vi "Update GUI (SubVI).vi"(11 "Data out":T1={"VI References"=[], "Addresses"=[], "Pilot"=FALSE, "DO Data"=[], "Access Restricted?"=FALSE, "Pilot Control References"=[], "CoPilot Control References"=[], "cRIO Config"=[], "datalog Q"=refnum, "PS_P"={"AI"=[], "DI"=[], "DO"=[], "Serial"=[], "CPU"={"Total Load"=[], "Interrupt Load"=[], "Total Physical"=0.0, "Free Physical"=0.0, "Primary Disk Capacity"=0.0, "Primary Disk Free"=0.0}, "Stop"=FALSE, "DO Channel"=[]}, "PS_S"={"AI"=[], "DI"=[], "DO"=[], "Serial"=[], "CPU"={"Total Load"=[], "Interrupt Load"=[], "Total Physical"=0.0, "Free Physical"=0.0, "Primary Disk Capacity"=0.0, "Primary Disk Free"=0.0}, "Stop"=FALSE, "DO Channel"=[]}, "IDE_P"={"AI"=[], "DI"=[], "DO"=[], "Serial"=[], "CPU"={"Total Load"=[], "Interrupt Load"=[], "Total Physical"=0.0, "Free Physical"=0.0, "Primary Disk Capacity"=0.0, "Primary Disk Free"=0.0}, "Stop"=FALSE, "DO Channel"=[]}, "IDE_S"={"AI"=[], "DI"=[], "DO"=[], "Serial"=[], "CPU"={"Total Load"=[], "Interrupt Load"=[], "Total Physical"=0.0, "Free Physical"=0.0, "Primary Disk Capacity"=0.0, "Primary Disk Free"=0.0}, "Stop"=FALSE, "DO Channel"=[]}, "PDE_P"={"AI"=[], "DI"=[], "DO"=[], "Serial"=[], "CPU"={"Total Load"=[], "Interrupt Load"=[], "Total Physical"=0.0, "Free Physical"=0.0, "Primary Disk Capacity"=0.0, "Primary Disk Free"=0.0}, "Stop"=FALSE, "DO Channel"=[]}, "PDE_S"={"AI"=[], "DI"=[], "DO"=[], "Serial"=[], "CPU"={"Total Load"=[], "Interrupt Load"=[], "Total Physical"=0.0, "Free Physical"=0.0, "Primary Disk Capacity"=0.0, "Primary Disk Free"=0.0}, "Stop"=FALSE, "DO Channel"=[]}, "GUI References"={"Control Names"=[], "Control References"=[]}, "GUI Data"=[], "TCP - Serial"=[], "TCP-Serial Q"=refnum, "TCP Serial Ref"=[], "Data Sets"=[], "Last Data"=[], "Alarm Data"=[], "DI Data"=[], "Ack Data"=[], "Buzzer Data"=[], "Pilot DO"=[], "Co-Pilot DO"=[], "System Down?"=FALSE, "Log Data"=[], "Update Array"=[], "MCC Data Log"=[], "MCC Data Not"=refnum, "Thruster control"=[refnum, refnum, refnum, refnum, refnum, refnum, refnum, refnum, refnum], "waga notifier out"=refnum, "Wago  log"=[], "Thruster Cont"=[0.0, 0.0, 0.0, 0.0, 0.0, 0.0, 0.0, 0.0, 0.0], "Cam Cont"=[FALSE, FALSE, FALSE, FALSE, FALSE, TRUE], "PDE_P TH Cont"={"COM 10"=0.0, "COM 11"=0.0, "COM 12"=0.0, "COM 13"=0.0}, "PDE_S TH Cont"={"COM 10"=0.0, "COM 11"=0.0, "COM 12"=0.0, "COM 13"=0.0}} {"cRIO Config"."AI"."Interface Data"."Timing"."sample mode" items=["Finite Samples"=10178, "Continuous Samples"=10123, "Hardware Timed Single Point"=12522]; "cRIO Config"."Async"."Interface Data"."Data"."Minor Frame Count" min=5 max=8 step=1}) -> (3 "Data out":T1={"VI References"=[], "Addresses"=[], "Pilot"=FALSE, "DO Data"=[], "Access Restricted?"=FALSE, "Pilot Control References"=[], "CoPilot Control References"=[], "cRIO Config"=[], "datalog Q"=refnum, "PS_P"={"AI"=[], "DI"=[], "DO"=[], "Serial"=[], "CPU"={"Total Load"=[], "Interrupt Load"=[], "Total Physical"=0.0, "Free Physical"=0.0, "Primary Disk Capacity"=0.0, "Primary Disk Free"=0.0}, "Stop"=FALSE, "DO Channel"=[]}, "PS_S"={"AI"=[], "DI"=[], "DO"=[], "Serial"=[], "CPU"={"Total Load"=[], "Interrupt Load"=[], "Total Physical"=0.0, "Free Physical"=0.0, "Primary Disk Capacity"=0.0, "Primary Disk Free"=0.0}, "Stop"=FALSE, "DO Channel"=[]}, "IDE_P"={"AI"=[], "DI"=[], "DO"=[], "Serial"=[], "CPU"={"Total Load"=[], "Interrupt Load"=[], "Total Physical"=0.0, "Free Physical"=0.0, "Primary Disk Capacity"=0.0, "Primary Disk Free"=0.0}, "Stop"=FALSE, "DO Channel"=[]}, "IDE_S"={"AI"=[], "DI"=[], "DO"=[], "Serial"=[], "CPU"={"Total Load"=[], "Interrupt Load"=[], "Total Physical"=0.0, "Free Physical"=0.0, "Primary Disk Capacity"=0.0, "Primary Disk Free"=0.0}, "Stop"=FALSE, "DO Channel"=[]}, "PDE_P"={"AI"=[], "DI"=[], "DO"=[], "Serial"=[], "CPU"={"Total Load"=[], "Interrupt Load"=[], "Total Physical"=0.0, "Free Physical"=0.0, "Primary Disk Capacity"=0.0, "Primary Disk Free"=0.0}, "Stop"=FALSE, "DO Channel"=[]}, "PDE_S"={"AI"=[], "DI"=[], "DO"=[], "Serial"=[], "CPU"={"Total Load"=[], "Interrupt Load"=[], "Total Physical"=0.0, "Free Physical"=0.0, "Primary Disk Capacity"=0.0, "Primary Disk Free"=0.0}, "Stop"=FALSE, "DO Channel"=[]}, "GUI References"={"Control Names"=[], "Control References"=[]}, "GUI Data"=[], "TCP - Serial"=[], "TCP-Serial Q"=refnum, "TCP Serial Ref"=[], "Data Sets"=[], "Last Data"=[], "Alarm Data"=[], "DI Data"=[], "Ack Data"=[], "Buzzer Data"=[], "Pilot DO"=[], "Co-Pilot DO"=[], "System Down?"=FALSE, "Log Data"=[], "Update Array"=[], "MCC Data Log"=[], "MCC Data Not"=refnum, "Thruster control"=[refnum, refnum, refnum, refnum, refnum, refnum, refnum, refnum, refnum], "waga notifier out"=refnum, "Wago  log"=[], "Thruster Cont"=[0.0, 0.0, 0.0, 0.0, 0.0, 0.0, 0.0, 0.0, 0.0], "Cam Cont"=[FALSE, FALSE, FALSE, FALSE, FALSE, TRUE], "PDE_P TH Cont"={"COM 10"=0.0, "COM 11"=0.0, "COM 12"=0.0, "COM 13"=0.0}, "PDE_S TH Cont"={"COM 10"=0.0, "COM 11"=0.0, "COM 12"=0.0, "COM 13"=0.0}} {"cRIO Config"."AI"."Interface Data"."Timing"."sample mode" items=["Finite Samples"=10178, "Continuous Samples"=10123, "Hardware Timed Single Point"=12522]; "cRIO Config"."Async"."Interface Data"."Data"."Minor Frame Count" min=5 max=8 step=1})   [LabVIEW 2021]
doc: "output from the c-RIO will be updated here with the help of the 2D string array mapping from the intilizle array. based on the mapping teh index of the controls will be got and its match with the reference index and data will be updated"
uses:
  Controls/Host - GUI Data Cluster.ctl
  Analog Output/Controls/AO JSON Data Cluster.ctl
  Analog Output/Controls/AO Interface Data Cluster.ctl
  Analog Output/Controls/AO Channel Configuration Cluster.ctl
  Analog Output/Controls/AO Timing Cluster.ctl
  Digital Output/Controls/DIO Configuration cluster.ctl
  Digital Output/Controls/DIO Interface Data.ctl
  Digital Output/SubVIs/Digital Dynamic Cluster.ctl
  Async JSON Cluster.ctl
  Async Interface Data Cluster.ctl
  Async Serial/Controls/Async Serial Configuration Cluster.ctl
  Async Serial/Controls/Async Frame Info Cluster.ctl
  Async Serial/Controls/Async Message Info Cluster.ctl
  Controls/Host Data Cluster.ctl
  Main Engine/Controls/Main Engine CPU Info.ctl
panel:
  out "error out 2":errorcluster
  out "error out":errorcluster
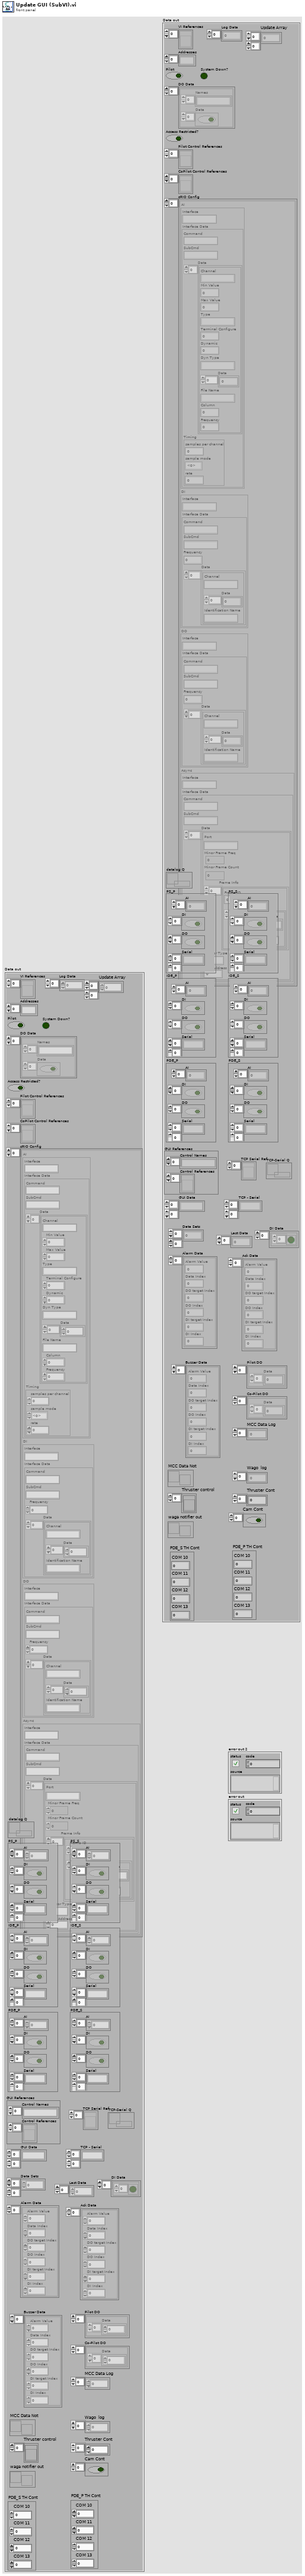
[diagram p1: front panel]
types:
  T1 = typedef "Host - GUI Data Cluster.ctl" = cluster{"VI References":refnum<vi>[], "Addresses":string[], "Pilot":bool, "DO Data":cluster{"Names":string[], "Data":bool[]}[], "Access Restricted?":bool, "Pilot Control References":refnum<vi>[], "CoPilot Control References":refnum<vi>[], "cRIO Config":cluster{"AI":T2, "DI":T6, "DO":T6, "Async":T9}[], "datalog Q":refnum<queue>, "PS_P":T14, "PS_S":T14, "IDE_P":T14, "IDE_S":T14, "PDE_P":T14, "PDE_S":T14, "GUI References":cluster{"Control Names":string[], "Control References":refnum<vi>[]}, "GUI Data":string[][], "TCP - Serial":string[][], "TCP-Serial Q":refnum<queue>, "TCP Serial Ref":refnum<vi>[], "Data Sets":dbl[][], "Last Data":dbl[], "Alarm Data":cluster{"Alarm Value":dbl, "Data Index":i32, "DO target Index":i32, "DO Index":i32, "DI target Index":i32, "DI Index":i32}[], "DI Data":cluster{bool[]}[], "Ack Data":cluster{"Alarm Value":dbl, "Data Index":i32, "DO target Index":i32, "DO Index":i32, "DI target Index":i32, "DI Index":i32}[], "Buzzer Data":cluster{"Alarm Value":dbl, "Data Index":i32, "DO target Index":i32, "DO Index":i32, "DI target Index":i32, "DI Index":i32}[], "Pilot DO":cluster{"Data":i32[]}[], "Co-Pilot DO":cluster{"Data":i32[]}[], "System Down?":bool, "Log Data":dbl[], "Update Array":i32[][], "MCC Data Log":dbl[], "MCC Data Not":refnum<notifier>, "Thruster control":refnum<vi>[], "waga notifier out":refnum<notifier>, "Wago  log":sgl[], "Thruster Cont":dbl[], "Cam Cont":bool[], "PDE_P TH Cont":cluster{"COM 10":dbl, "COM 11":dbl, "COM 12":dbl, "COM 13":dbl}, "PDE_S TH Cont":cluster{"COM 10":dbl, "COM 11":dbl, "COM 12":dbl, "COM 13":dbl}}
  T2 = typedef "AO JSON Data Cluster.ctl" = cluster{"Interface":string, "Interface Data":T3}
  T3 = typedef "AO Interface Data Cluster.ctl" = cluster{"Command":string, "SubCmd":string, "Data":T4[], "Timing":T5}
  T4 = typedef "AO Channel Configuration Cluster.ctl" = cluster{"Channel":string, "Min Value":dbl, "Max Value":dbl, "Type":string, "Terminal Configure":u16, "Dynamic":u8, "Dyn Type":string, "Data":dbl[], "File Name":string, "Column":i32, "Frequency":dbl}
  T5 = typedef "AO Timing Cluster.ctl" = cluster{"samples per channel":i32, "sample mode":i32, "rate":dbl}
  T6 = typedef "DIO Configuration cluster.ctl" = cluster{"Interface":string, "Interface Data":T7}
  T7 = typedef "DIO Interface Data.ctl" = cluster{"Command":string, "SubCmd":string, "Frequency":u16, "Data":T8[]}
  T8 = typedef "Digital Dynamic Cluster.ctl" = cluster{"Channel":string, "Data":u8[], "Identification Name":string}
  T9 = typedef "Async JSON Cluster.ctl" = cluster{"Interface":string, "Interface Data":T10}
  T10 = typedef "Async Interface Data Cluster.ctl" = cluster{"Command":string, "SubCmd":string, "Data":T11[]}
  T11 = typedef "Async Serial Configuration Cluster.ctl" = cluster{"Port":string, "Minor Frame Freq":u16, "Minor Frame Count":u16, "Frame Info":T12[], "Sensor Type":u16, "OIM Address":u16}
  T12 = typedef "Async Frame Info Cluster.ctl" = cluster{"Frame ID":u16, "Message Info":T13[]}
  T13 = typedef "Async Message Info Cluster.ctl" = cluster{"Message":u8[], "Message Name":string}
  T14 = typedef "Host Data Cluster.ctl" = cluster{"AI":dbl[], "DI":bool[], "DO":bool[], "Serial":string[][], "CPU":T15, "Stop":bool, "DO Channel":string[]}
  T15 = typedef "Main Engine CPU Info.ctl" = cluster{"Total Load":u32[], "Interrupt Load":u32[], "Total Physical":dbl, "Free Physical":dbl, "Primary Disk Capacity":dbl, "Primary Disk Free":dbl}
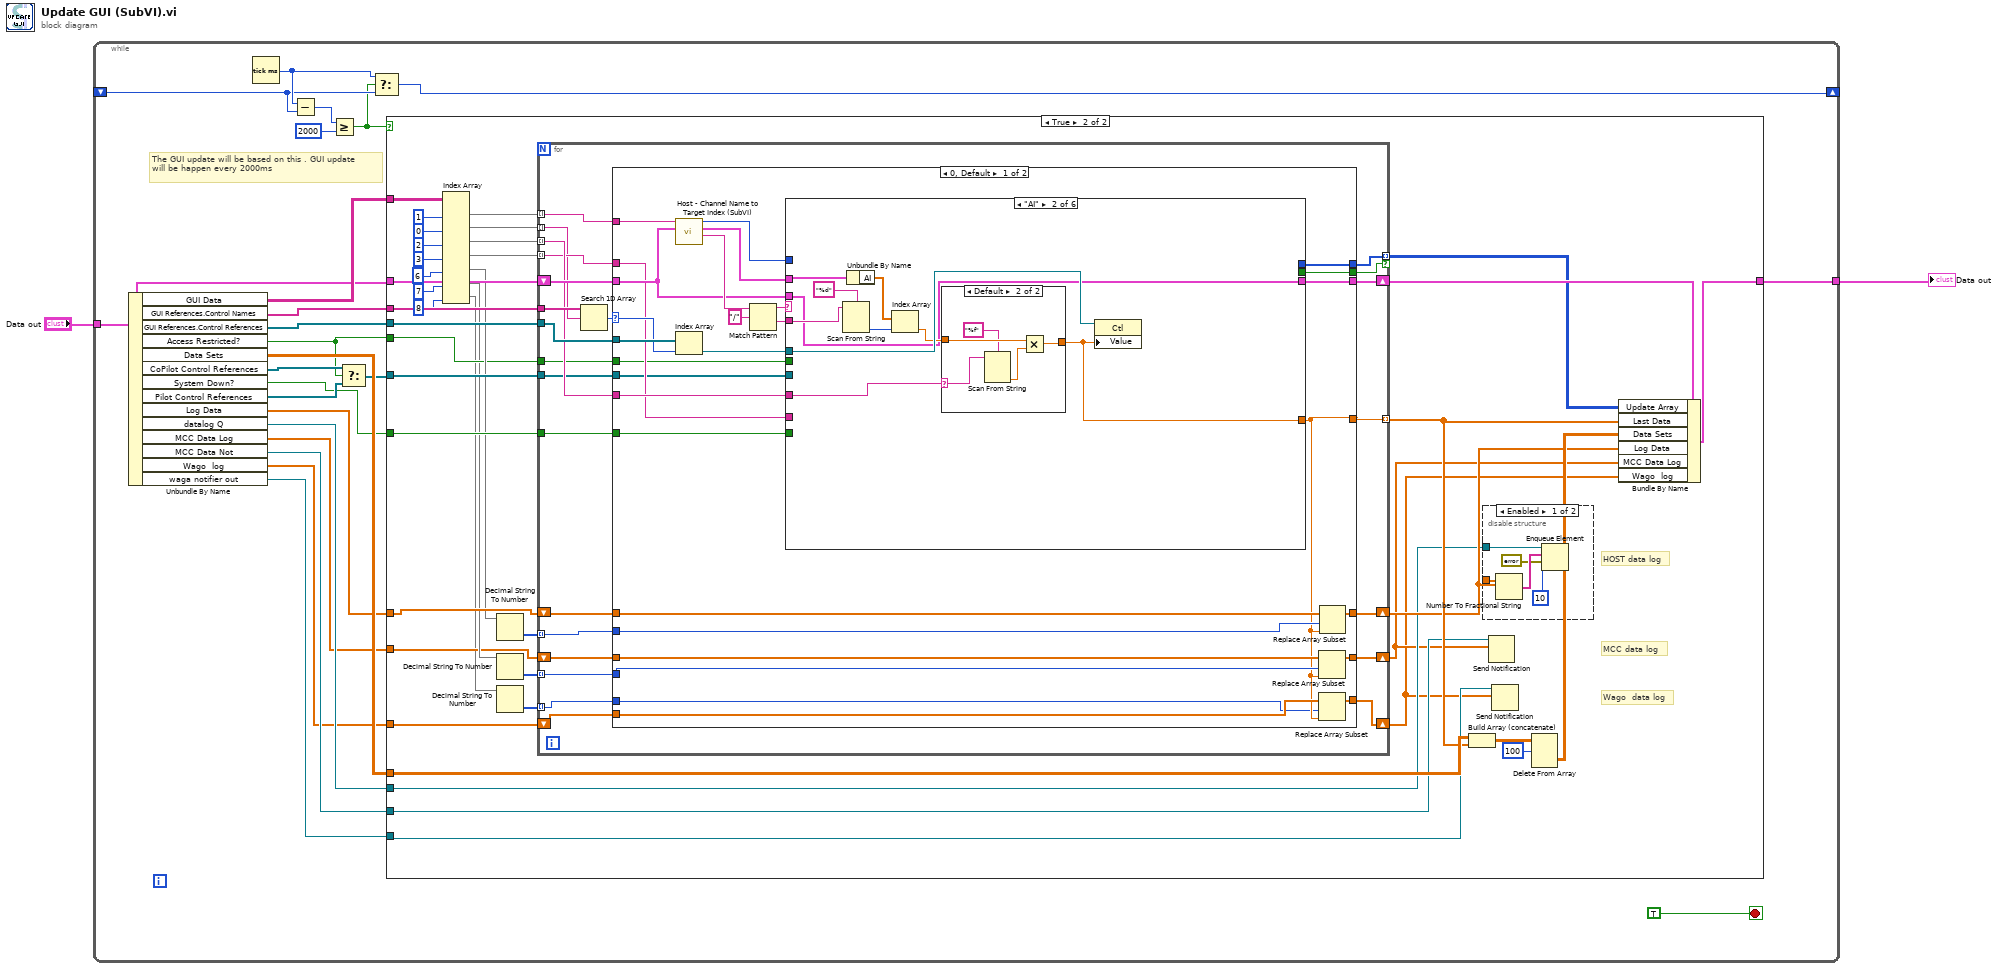
[diagram p0: block diagram]
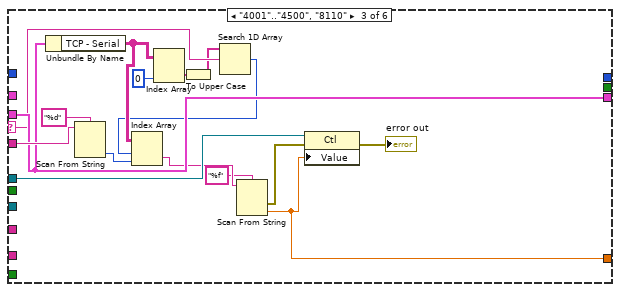
[diagram p6: hidden frame]
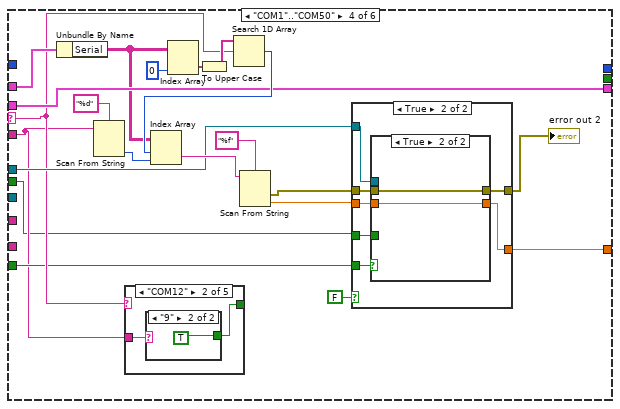
[diagram p7: hidden frame]
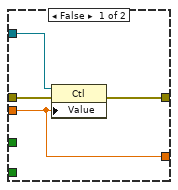
[diagram p8: hidden frame]
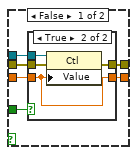
[diagram p9: hidden frame]
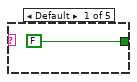
[diagram p11: hidden frame]
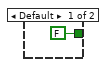
[diagram p12: hidden frame]
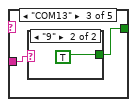
[diagram p13: hidden frame]
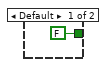
[diagram p14: hidden frame]
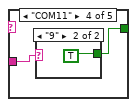
[diagram p15: hidden frame]
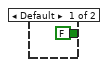
[diagram p16: hidden frame]
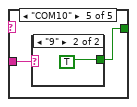
[diagram p17: hidden frame]
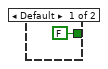
[diagram p18: hidden frame]
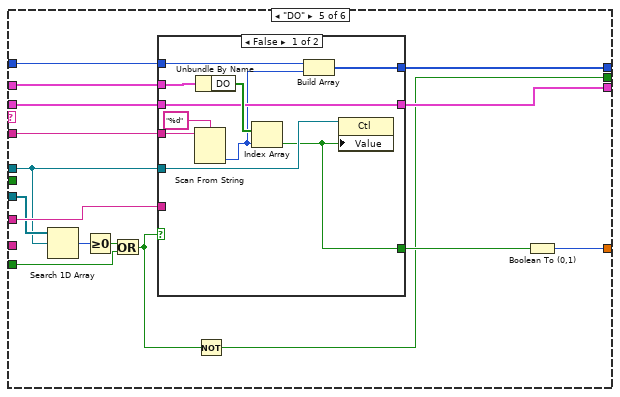
[diagram p19: hidden frame]
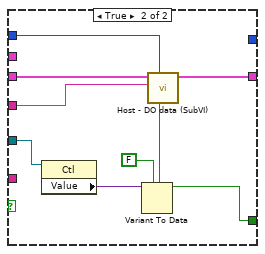
[diagram p20: hidden frame]
diagram:
  n1 = while {
    tunnel: "Data out" -> [w23]
    shift-right: [w17] -> _
    shift-left: _ -> [w18]
    tunnel: [w14] -> w2
    stop <- TRUE stop-if-true
    # "The GUI update will be based on this . GUI update   \nwill be happen every 2000ms"
    n2 = Unbundle By Name(w23) -> ("GUI Data"=w26:string[][], "GUI References.Control Names"=w25:string[], "GUI References.Control References"=w24:refnum<vi>[], "Access Restricted?"=w7:bool, "Data Sets"=w15:dbl[][], "CoPilot Control References"=w12:refnum<vi>[], "System Down?"=w10:bool, "Pilot Control References"=w11:refnum<vi>[], "Log Data"=w9:dbl[], "datalog Q"=w8:refnum<queue>, "MCC Data Log"=w6:dbl[], "MCC Data Not"=w5:refnum<notifier>, "Wago  log"=w4:sgl[], "waga notifier out"=w3:refnum<notifier>)
    n3 = Tick Count (ms)() -> (millisecond timer value=w19:u32)
    n4 = Subtract(x=w19, y=w18) -> (x-y=w21:u32)
    n5 = Greater Or Equal?(x=w21, y=u32 2000) -> (x >= y?=w16:bool)
    n6 = Select(t=w12, s=w7, f=w11) -> (s? t:f=w13:refnum<vi>[])
    n7 = Select(t=w19, s=w16, f=w18) -> (s? t:f=w17:u32)
    n8 = case shown="True" w16 {
      tunnel: w26 -> [_ w68]
      tunnel: w25 -> [_ w65]
      tunnel: w24 -> [_ w64]
      tunnel: w23 -> [w27 w63]
      tunnel: [w27 w51] -> w14
      tunnel: w15 -> [_ w58]
      tunnel: w13 -> [_ w49]
      tunnel: w10 -> [_ w48]
      tunnel: w9 -> [_ w46]
      tunnel: w8 -> [_ w42]
      tunnel: w7 -> [_ w40]
      tunnel: w6 -> [_ w36]
      tunnel: w5 -> [_ w35]
      tunnel: w4 -> [_ w30]
      tunnel: w3 -> [_ w29]
      frame False {
      }
      frame True {
        # "Wago  data log"
        # "HOST data log"
        # "MCC data log"
        n9 = Index Array(array=w68, index (col) #1=1 ("index (col)"), index (col) #2=0 ("index (col)"), index (col) #3=2 ("index (col)"), index (col) #4=3 ("index (col)"), index (col) #5=6 ("index (col)"), index (col) #6=7 ("index (col)"), index (col) #7=8 ("index (col)")) -> (element #1=w66:string[], element #2=w61:string[], element #3=w59:string[], element #4=w56:string[], element #5=w45:string[], element #6=w38:string[], element #7=w32:string[])  [unwired: 7 in]
        n10 = Decimal String To Number(string=w45) -> (number=w44:i32[])  [unwired: 2 in, 1 out]
        n11 = Decimal String To Number(string=w38) -> (number=w37:i32[])  [unwired: 2 in, 1 out]
        n12 = Decimal String To Number(string=w32) -> (number=w31:i32[])  [unwired: 2 in, 1 out]
        n13 = for {
          tunnel: w66 -> [w96] mode=indexing
          tunnel: w65 -> [w97]
          tunnel: w64 -> [w94]
          tunnel: w61 -> [w87] mode=indexing
          tunnel: w59 -> [w92] mode=indexing
          shift-right: [w91] -> w53
          shift-left: w63 -> [w93]
          tunnel: [w90] -> w50 mode=indexing
          tunnel: w56 -> [w89] mode=indexing
          tunnel: w49 -> [w88]
          tunnel: w48 -> [w86]
          tunnel: w44 -> [w84] mode=indexing
          shift-right: [w83] -> w43
          shift-left: w46 -> [w85]
          tunnel: [w82] -> w41 mode=indexing if=w81
          tunnel: w40 -> [w80]
          tunnel: w37 -> [w79] mode=indexing
          shift-right: [w77] -> w34
          shift-left: w36 -> [w78]
          tunnel: w31 -> [w76] mode=indexing
          shift-right: [w74] -> w28
          shift-left: w30 -> [w75]
          n14 = Search 1D Array(1D array=w97, element=w87) -> (index of element=w95:i32)  [unwired: 1 in]
          n15 = case shown="0, Default" w95 {
            selector: w95 -> [w124 _]
            tunnel: w96 -> [w126 _]
            tunnel: w94 -> [w125 _]
            tunnel: w93 -> [w116 w274]
            tunnel: w92 -> [w117 _]
            tunnel: [w114 w274] -> w91
            tunnel: [w99 _] -> w90
            tunnel: w89 -> [w113 _]
            tunnel: w88 -> [w112 _]
            tunnel: w86 -> [w111 _]
            tunnel: w84 -> [w110 _]
            tunnel: w85 -> [w105 w273]
            tunnel: [w109 w273] -> w83
            tunnel: [w108 _] -> w82
            tunnel: [w107 _] -> w81
            tunnel: w80 -> [w106 _]
            tunnel: w79 -> [w104 _]
            tunnel: w78 -> [w103 w272]
            tunnel: [w102 w272] -> w77
            tunnel: w76 -> [w98 _]
            tunnel: w75 -> [w101 w271]
            tunnel: [w100 w271] -> w74
            frame 0, Default {
              n16 = call "Host - Channel Name to Target Index (SubVI).vi"("Data in"=w116, "Channel In"=w126) -> ("Channel Out"=w121:string, "Target Data"=w123:T14, "Target Index"=w115:i32)  [unwired: 7 in]
              n17 = Index Array(array=w125, index=w124) -> (element=w118:refnum<vi>)
              n18 = Match Pattern(string=w121, regular expression="/") -> (before substring=w120:string, after substring=w119:string)  [unwired: 1 in, 2 out]
              n19 = case shown="\"AI\"" w120 {
                selector: w120 -> [_ _ w146 w165 _ _]
                tunnel: w123 -> [_ w135 _ w172 w237 w266]
                tunnel: w119 -> [_ w137 w159 w163 w238 w267]
                tunnel: w118 -> [_ w132 w157 w169 w229 w265]
                tunnel: w117 -> [_ w130 _ _ w236 w264]
                tunnel: w116 -> [w127 w129 w156 w173 w235 w259]
                tunnel: w115 -> [_ _ _ _ w234 _]
                tunnel: [w127 w129 w156 w173 w233 w259] -> w114
                tunnel: [_ w128 w145 w160 w231 w258] -> w99
                tunnel: w113 -> [_ _ _ _ _ _]
                tunnel: w112 -> [_ _ _ _ w230 _]
                tunnel: w111 -> [_ _ _ w164 w226 _]
                tunnel: [_ _ _ _ w225 _] -> w108
                tunnel: [_ _ _ _ w223 _] -> w107
                tunnel: w106 -> [_ _ _ w162 _ _]
                frame Default {
                }
                frame "AI" {
                  n20 = Scan From String(format string="%d", input string=w137) -> (output 1=w133:i32)  [unwired: 3 in, 3 out]
                  n21 = Unbundle By Name(w135) -> ("AI"=w134:dbl[])
                  n22 = Index Array(array=w134, index=w133) -> (element=w131:dbl)
                  n23 = case shown="Default" w130 {
                    selector: w130 -> [_ w140]
                    tunnel: w131 -> [w138 w143]
                    tunnel: [w138 w142] -> w128
                    frame "" {
                    }
                    frame Default {
                      n24 = Scan From String(format string="%f", input string=w140) -> (output 1=w139:dbl)  [unwired: 3 in, 3 out]
                      n25 = Multiply(x=w143, y=w139) -> (x*y=w142:dbl)
                    }
                  }
                  n26 = property class="Ctl"(reference=w132, "Value"=w128) -> ()  [unwired: 1 in, 2 out]
                }
                frame "4001".."4500", "8110" {
                  n27 = Unbundle By Name(w156) -> ("TCP - Serial"=w153:string[][])
                  n28 = Scan From String(format string="%d", input string=w159) -> (output 1=w151:i32)  [unwired: 3 in, 3 out]
                  n29 = Index Array(array=w153, index (col)=0 ("disabled index (col)")) -> (element=w154:string[])  [unwired: 1 in]
                  n30 = To Upper Case(1:w154) -> (0:w144:string[])
                  n31 = Search 1D Array(1D array=w144, element=w146) -> (index of element=w152:i32)  [unwired: 1 in]
                  n32 = Index Array(array=w153, index (row)=w152, index (col)=w151) -> (element=w150:string)
                  n33 = Scan From String(format string="%f", input string=w150) -> (error out=w148:errorcluster, output 1=w145:dbl)  [unwired: 3 in, 2 out]
                  n34 = property class="Ctl"(reference=w157, error in=w148, "Value"=w145) -> (error out=→"error out":errorcluster)  [unwired: 1 out]
                }
                frame "COM1".."COM50" {
                  n35 = Unbundle By Name(w172) -> ("Serial"=w171:string[][])
                  n36 = Scan From String(format string="%d", input string=w163) -> (output 1=w176:i32)  [unwired: 3 in, 3 out]
                  n37 = case shown="\"COM12\"" w165 {
                    tunnel: [FALSE ("Access Restricted?") w207 w212 w216 w220] -> _
                    tunnel: w163 -> [_ w208 w211 w215 w219]
                    frame Default {
                    }
                    frame "COM12" {
                      n38 = case shown="\"9\"" w208 {
                        tunnel: [FALSE ("Access Restricted?") TRUE ("Access Restricted?")] -> w207
                        frame Default {
                        }
                        frame "9" {
                        }
                      }
                    }
                    frame "COM13" {
                      n39 = case shown="\"9\"" w211 {
                        tunnel: [FALSE ("Access Restricted?") TRUE ("Access Restricted?")] -> w212
                        frame Default {
                        }
                        frame "9" {
                        }
                      }
                    }
                    frame "COM11" {
                      n40 = case shown="\"9\"" w215 {
                        tunnel: [FALSE ("Access Restricted?") TRUE ("Access Restricted?")] -> w216
                        frame Default {
                        }
                        frame "9" {
                        }
                      }
                    }
                    frame "COM10" {
                      n41 = case shown="\"9\"" w219 {
                        tunnel: [FALSE ("Access Restricted?") TRUE ("Access Restricted?")] -> w220
                        frame Default {
                        }
                        frame "9" {
                        }
                      }
                    }
                  }
                  n42 = Index Array(array=w171, index (col)=0 ("disabled index (col)")) -> (element=w178:string[])  [unwired: 1 in]
                  n43 = To Upper Case(1:w178) -> (0:w170:string[])
                  n44 = Search 1D Array(1D array=w170, element=w165) -> (index of element=w177:i32)  [unwired: 1 in]
                  n45 = Index Array(array=w171, index (row)=w177, index (col)=w176) -> (element=w175:string)
                  n46 = Scan From String(format string="%f", input string=w175) -> (error out=w167:errorcluster, output 1=w168:dbl)  [unwired: 3 in, 2 out]
                  n47 = case shown="True" FALSE {
                    tunnel: w169 -> [w182 w191]
                    tunnel: w168 -> [w181 w190]
                    tunnel: w167 -> [w184 w189]
                    tunnel: [w183 w188] -> w166
                    tunnel: w164 -> [_ w187]
                    tunnel: w162 -> [_ w186]
                    tunnel: [w181 w185] -> w160
                    frame False {
                      n48 = property class="Ctl"(reference=w182, error in=w184, "Value"=w181) -> (error out=w183:errorcluster)  [unwired: 1 out]
                    }
                    frame True {
                      n49 = case shown="True" w187 {
                        tunnel: w191 -> [w197 _]
                        tunnel: w190 -> [w196 w204]
                        tunnel: w189 -> [w195 w205]
                        tunnel: [w194 w205] -> w188
                        tunnel: w186 -> [w193 _]
                        tunnel: [w192 w204] -> w185
                        frame False {
                          n50 = case shown="True" w193 {
                            tunnel: w197 -> [_ w203]
                            tunnel: w196 -> [w198 w200]
                            tunnel: w195 -> [w199 w202]
                            tunnel: [w199 w201] -> w194
                            tunnel: [w198 w200] -> w192
                            frame False {
                            }
                            frame True {
                              n51 = property class="Ctl"(reference=w203, error in=w202, "Value"=w200) -> (error out=w201:errorcluster)  [unwired: 1 out]
                            }
                          }
                        }
                        frame True {
                        }
                      }
                    }
                  }
                  "error out 2" <- w166
                }
                frame "DO" {
                  n52 = Search 1D Array(1D array=w230, element=w229) -> (index of element=w228:i32)  [unwired: 1 in]
                  n53 = Greater Or Equal To 0?(x=w228) -> (x >= 0?=w227:bool)
                  n54 = Or(x=w227, y=w226) -> (x .or. y?=w224:bool)
                  n55 = case shown="False" w224 {
                    tunnel: w238 -> [w248 w256]
                    tunnel: w237 -> [w246 _]
                    tunnel: w229 -> [w244 w255]
                    tunnel: w236 -> [_ _]
                    tunnel: w235 -> [w243 w250]
                    tunnel: w234 -> [w241 w249]
                    tunnel: [w243 w252] -> w233
                    tunnel: [w242 w251] -> w232
                    tunnel: [w239 _] -> w225
                    frame False {
                      n56 = Scan From String(format string="%d", input string=w248) -> (output 1=w240:i32)  [unwired: 3 in, 3 out]
                      n57 = Unbundle By Name(w246) -> ("DO"=w245:bool[])
                      n58 = Index Array(array=w245, index=w240) -> (element=w242:bool)
                      n59 = Build Array(w241, w240) -> (w239:i32[])
                      n60 = property class="Ctl"(reference=w244, "Value"=w242) -> ()  [unwired: 1 in, 2 out]
                    }
                    frame True {
                      n61 = property class="Ctl"(reference=w255) -> ("Value"=w254:variant)  [unwired: 1 in, 2 out]
                      n62 = Variant To Data(type=FALSE, Variant=w254) -> (data=w251:bool)  [unwired: 1 in, 1 out]
                      n63 = call "Host - DO data (SubVI).vi"("New Data"=w251, "Target Index"=w249, "Channel Index"=w256, "Data in"=w250) -> ("Data out"=w252:T1)  [unwired: 7 in]
                    }
                  }
                  n64 = Not(x=w224) -> (.not. x?=w223:bool)
                  n65 = Boolean To (0,1)(Boolean=w232) -> (0, 1=w231:i16)
                }
                frame "DI" {
                  n66 = Scan From String(format string="%d", input string=w267) -> (output 1=w261:i32)  [unwired: 3 in, 3 out]
                  n67 = Unbundle By Name(w266) -> ("DI"=w262:bool[])
                  n68 = Index Array(array=w262, index=w261) -> (element=w260:bool)
                  n69 = case shown="\"-\"" w264 {
                    tunnel: w260 -> [w268 w270]
                    tunnel: [w268 w269] -> w257
                    frame Default {
                    }
                    frame "-" {
                      n70 = Not(x=w270) -> (.not. x?=w269:bool)
                    }
                  }
                  n71 = property class="Ctl"(reference=w265, "Value"=w257) -> ()  [unwired: 1 in, 2 out]
                  n72 = Boolean To (0,1)(Boolean=w257) -> (0, 1=w258:i16)
                }
              }
              n73 = Replace Array Subset(array=w103, new element=w99, index=w104) -> (w102:dbl[])
              n74 = Replace Array Subset(array=w101, new element=w99, index=w98) -> (w100:sgl[])
              n75 = Replace Array Subset(array=w105, new element=w99, index=w110) -> (w109:dbl[])
            }
            frame -1 {
            }
          }
        }
        n76 = Build Array (concatenate)(w58, w50) -> (w55:dbl[][])
        n77 = disable-structure shown="Enabled" {
          disable-tunnel: w43 -> [w72 _]
          disable-tunnel: w42 -> [w71 _]
          frame Enabled {
            n78 = Number To Fractional String(number=w72) -> (F-format string=w73:string[])  [unwired: 3 in]
            n79 = Enqueue Element(queue=w71, element=w73, timeout in ms (-1)=10, error in (no error)=errorcluster {"status"=FALSE, "code"=0, "source"=""}) -> ()  [unwired: 3 out]
          }
          frame Disabled {
          }
        }
        n80 = Send Notification(notification=w34, notifier=w35) -> ()  [unwired: 1 in, 2 out]
        n81 = Send Notification(notification=w28, notifier=w29) -> ()  [unwired: 1 in, 2 out]
        n82 = Delete From Array(array=w55, length=100) -> (deleted portion=w52:dbl[][])  [unwired: 2 in, 1 out]
        n83 = Bundle By Name(cluster=w53, "Update Array"=w41, "Last Data"=w50, "Data Sets"=w52, "Log Data"=w43, "MCC Data Log"=w34, "Wago  log"=w28) -> (w51:T1)
      }
    }
  }
  "Data out" <- w2
